vi "Set Cell Color and Border.vi"(1 "Border edges":T2={"Left   "=TRUE, "Right"=TRUE, "Top"=TRUE, "Bottom"=TRUE, "All"=FALSE}, 2 "Border style":T1, 4 "Fill Color":u32(colorbox), 5 "Border Color":u32(colorbox), 6 "Apply Fill":bool, 7 "Apply Border":bool, 8 "error in (no error)":errorcluster, 9 "End Cell Address":string, 10 "Start Cell Address":string, 11 "Report Ref In":T3) -> (0 "error out":errorcluster, 3 "Report Ref Out":T3)   [LabVIEW 2026, in "XCel Report Engine.lvlib"]
uses:
  XCel Report Engine.lvlib
  Controls/Report Ref.ctl
  Controls/Border edges.ctl
  Controls/Border style.ctl
  C:/Users/m.santucci/Documents/ChatGPT/LV_REPORT_ENGINE/.net/src/XCelReportEngine/bin/Release/net48/XCelReportEngine.dll
  .net/src/XCelReportEngine/bin/Release/net48/XCelReportEngine.dll
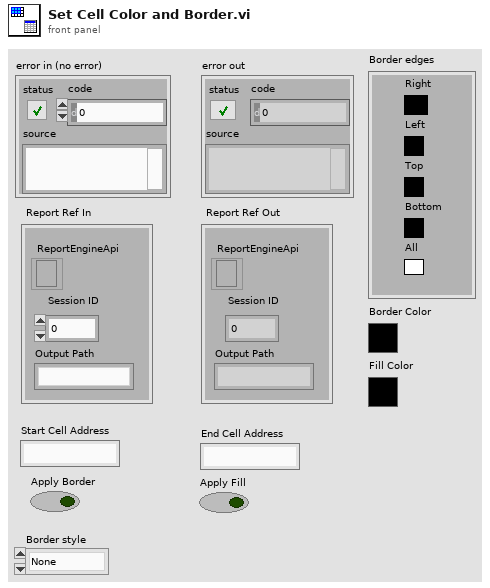
[diagram p1: front panel]
types:
  T1 = typedef "XCel Report Engine.lvlib/Border style.ctl" = enum16{"None", "Thin", "Medium", "Thick", "Double", "Dashed", "Dotted"}
  T2 = typedef "XCel Report Engine.lvlib/Border edges.ctl" = cluster{"Left   ":bool, "Right":bool, "Top":bool, "Bottom":bool, "All":bool}
  T3 = typedef "XCel Report Engine.lvlib/Report Ref.ctl" = cluster{"Session ID":i32, "Output Path":string, "ReportEngineApi":refnum<k24>}
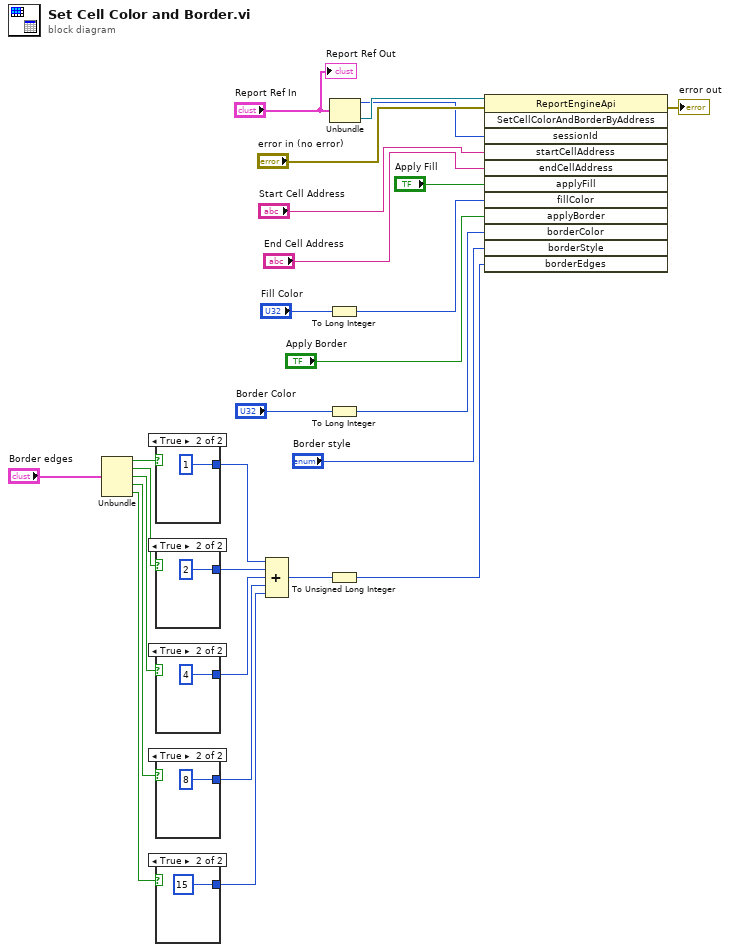
[diagram p0: block diagram]
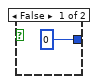
[diagram p2: hidden frame]
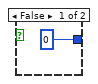
[diagram p3: hidden frame]
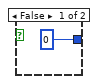
[diagram p4: hidden frame]
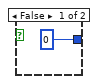
[diagram p5: hidden frame]
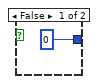
[diagram p6: hidden frame]
diagram:
  n1 = Unbundle("Border edges") -> ("Left"=w17:bool, "Right"=w16:bool, "Top"=w15:bool, "Bottom"=w14:bool, "All"=w13:bool)
  n2 = case shown="True" w17 {
    tunnel: [0 1] -> w12
    frame False {
    }
    frame True {
    }
  }
  n3 = case shown="True" w16 {
    tunnel: [0 2] -> w11
    frame False {
    }
    frame True {
    }
  }
  n4 = case shown="True" w15 {
    tunnel: [0 4] -> w10
    frame False {
    }
    frame True {
    }
  }
  n5 = case shown="True" w14 {
    tunnel: [0 8] -> w9
    frame False {
    }
    frame True {
    }
  }
  n6 = case shown="True" w13 {
    tunnel: [0 15] -> w8
    frame False {
    }
    frame True {
    }
  }
  n7 = Compound Arithmetic op=ADD(w12, w11, w10, w9, w8) -> (w6:i32)
  n8 = To Long Integer(number="Fill Color") -> (32bit integer=w1:i32)
  n9 = To Long Integer(number="Border Color") -> (32bit integer=w2:i32)
  n10 = To Unsigned Long Integer(number=w6) -> (unsigned 32bit integer=w5:u32)
  n11 = Unbundle("Report Ref In") -> ("Session ID"=w23:i32, "ReportEngineApi"=w26:refnum<k24>)  [unwired: 1 out]
  n12 = invoke class="ReportEngineApi" method="SetCellColorAndBorderByAddress"(reference=w26, error in="error in (no error)", "sessionId"=w23, "startCellAddress"="Start Cell Address", "endCellAddress"="End Cell Address", "applyFill"="Apply Fill", "fillColor"=w1, "applyBorder"="Apply Border", "borderColor"=w2, "borderStyle"="Border style", "borderEdges"=w5) -> (error out=→"error out":errorcluster)  [unwired: 1 in, 11 out]
  "Report Ref Out" <- "Report Ref In"
